vi "Operation.vi"(8 "Error In":errorcluster, 11 "Divide in":refnum<class "Divide.lvclass">) -> (0 "Error Out":errorcluster, 2 "C":dbl, 3 "Divide out":refnum<class "Divide.lvclass">)   [LabVIEW 2023, in "Divide.lvclass"]
doc: "The VI performs the division operation for two numbers and displays the output."
uses:
  Divide.lvclass
  Divide.lvclass/Divide.ctl
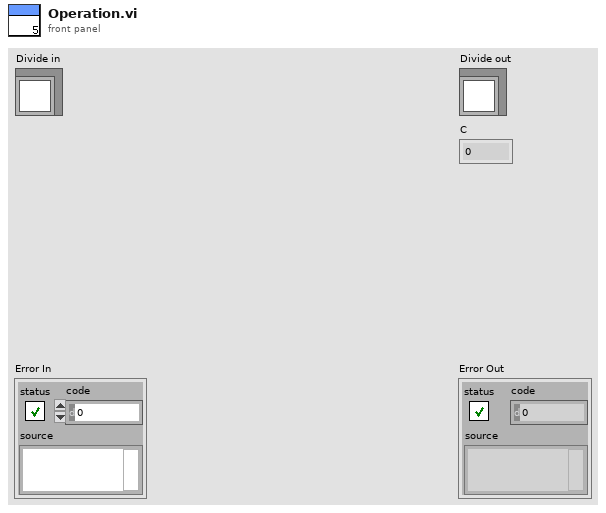
[diagram p1: front panel]
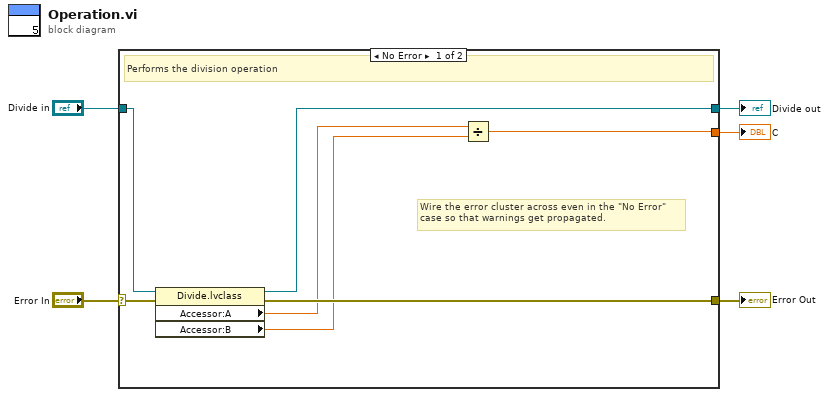
[diagram p0: block diagram]
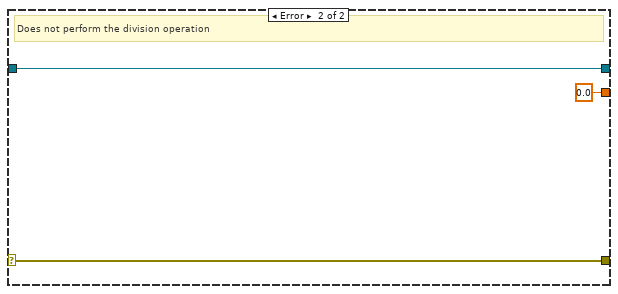
[diagram p2: hidden frame]
diagram:
  n1 = case shown="No Error" "Error In" {
    selector: "Error In" -> [w12 w15]
    tunnel: [w10 w15] -> w4
    tunnel: [w6 w14] -> w2
    tunnel: "Divide in" -> [w9 w14]
    tunnel: [w11 0.0] -> w1
    frame No Error {
      # "Wire the error cluster across even in the \"No Error\"\ncase so that warnings get propagated."
      # "Performs the division operation"
      n2 = property class="Divide.lvclass"(reference=w9, error in=w12) -> (reference out=w6:refnum<class "Divide.lvclass">, error out=w10:errorcluster, "Accessor:A"=w8:dbl, "Accessor:B"=w7:dbl)
      n3 = Divide(x=w8, y=w7) -> (x/y=w11:dbl)
    }
    frame Error {
      # "Does not perform the division operation"
    }
  }
  "Error Out" <- w4
  "Divide out" <- w2
  "C" <- w1
